vi "Set Property.vi"(0 "Filter in":refnum<class "Filter.lvclass">, 5 "Property":string, 7 "Value":dbl, 11 "error in (no error)":errorcluster) -> (4 "Filter out":refnum<class "Filter.lvclass">, 15 "error out":errorcluster)   [LabVIEW 2020, in "Filter.lvclass"]
uses:
  Filter.lvclass
  Filter.lvclass/Filter.ctl
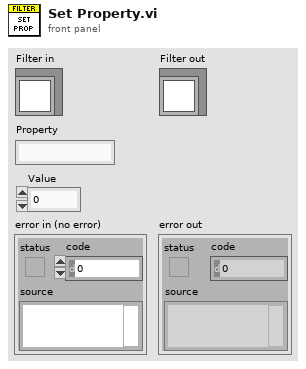
[diagram p1: front panel]
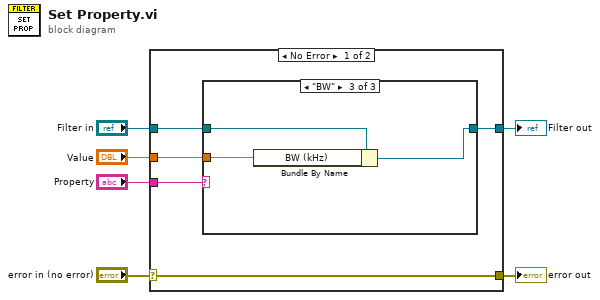
[diagram p0: block diagram]
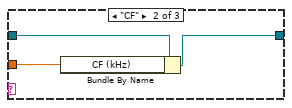
[diagram p3: hidden frame]
diagram:
  n1 = case shown="No Error" "error in (no error)" {
    selector: "error in (no error)" -> [w11 w20]
    tunnel: [w11 w20] -> w5
    tunnel: [w9 w19] -> w3
    tunnel: "Filter in" -> [w10 w19]
    tunnel: "Property" -> [w8 _]
    tunnel: "Value" -> [w7 _]
    frame No Error {
      n2 = case shown="\"BW\"" w8 {
        tunnel: w10 -> [w12 w15 w18]
        tunnel: w7 -> [_ w14 w17]
        tunnel: [w12 w13 w16] -> w9
        frame "False", Default {
        }
        frame "CF" {
          n3 = Bundle By Name(cluster=w15, "CF (kHz)"=w14) -> (w13:refnum<class "Filter.lvclass">)
        }
        frame "BW" {
          n4 = Bundle By Name(cluster=w18, "BW (kHz)"=w17) -> (w16:refnum<class "Filter.lvclass">)
        }
      }
    }
    frame Error {
    }
  }
  "error out" <- w5
  "Filter out" <- w3
